vi "SP_REJECTION_Count_DayWise.vi"(8 "error in (no error)":errorcluster) -> (0 "error out":errorcluster)   [LabVIEW 2017]
uses:
  <vilib>/Math Plots/3D Math Plots/3D Pie/3D Pie XCtrl/3D Pie.xctl
  <vilib>/addons/database/Connection.llb/DB Tools Open Connec (Path).vi
  <vilib>/addons/database/Connection.llb/Conn Execute.vi
  <vilib>/addons/database/Recordset.llb/Rec Fetch Recordset Data (R).vi
  <vilib>/addons/database/Recordset.llb/Rec Destroy - Connection.vi
  <vilib>/Math Plots/3D Math Plots/3D Pie/3D Pie Datatype/Public/Plot Helper (Vector).vi
  <vilib>/addons/database/NI_Database_API.lvlib
  <vilib>/Math Plots/3D Math Plots/3D Pie/3D Pie Datatype/3D Pie Datatype.lvclass
panel:
  out "Station list":string[](array[string])
  out "Station size":i32
  in  "Tab Control":enum32{"Data", "Graph"}(tab)
  out "Table":string[][](table)
  out "3D Pie":refnum<class "3D Plot Datatype.lvclass">[](xcontrol)
  in  "To Date":timestamp format="%<%Y-%m-%d>T"
  out "Station Count":i32
  in  "Cancel Button - Archive":bool
  in  "Download 2":bool
  in  "Get Rport 2":bool
  in  "Shift":string(combo)
  in  "Station":string(combo)
  in  "From Date":timestamp format="%<%Y-%m-%d>T"
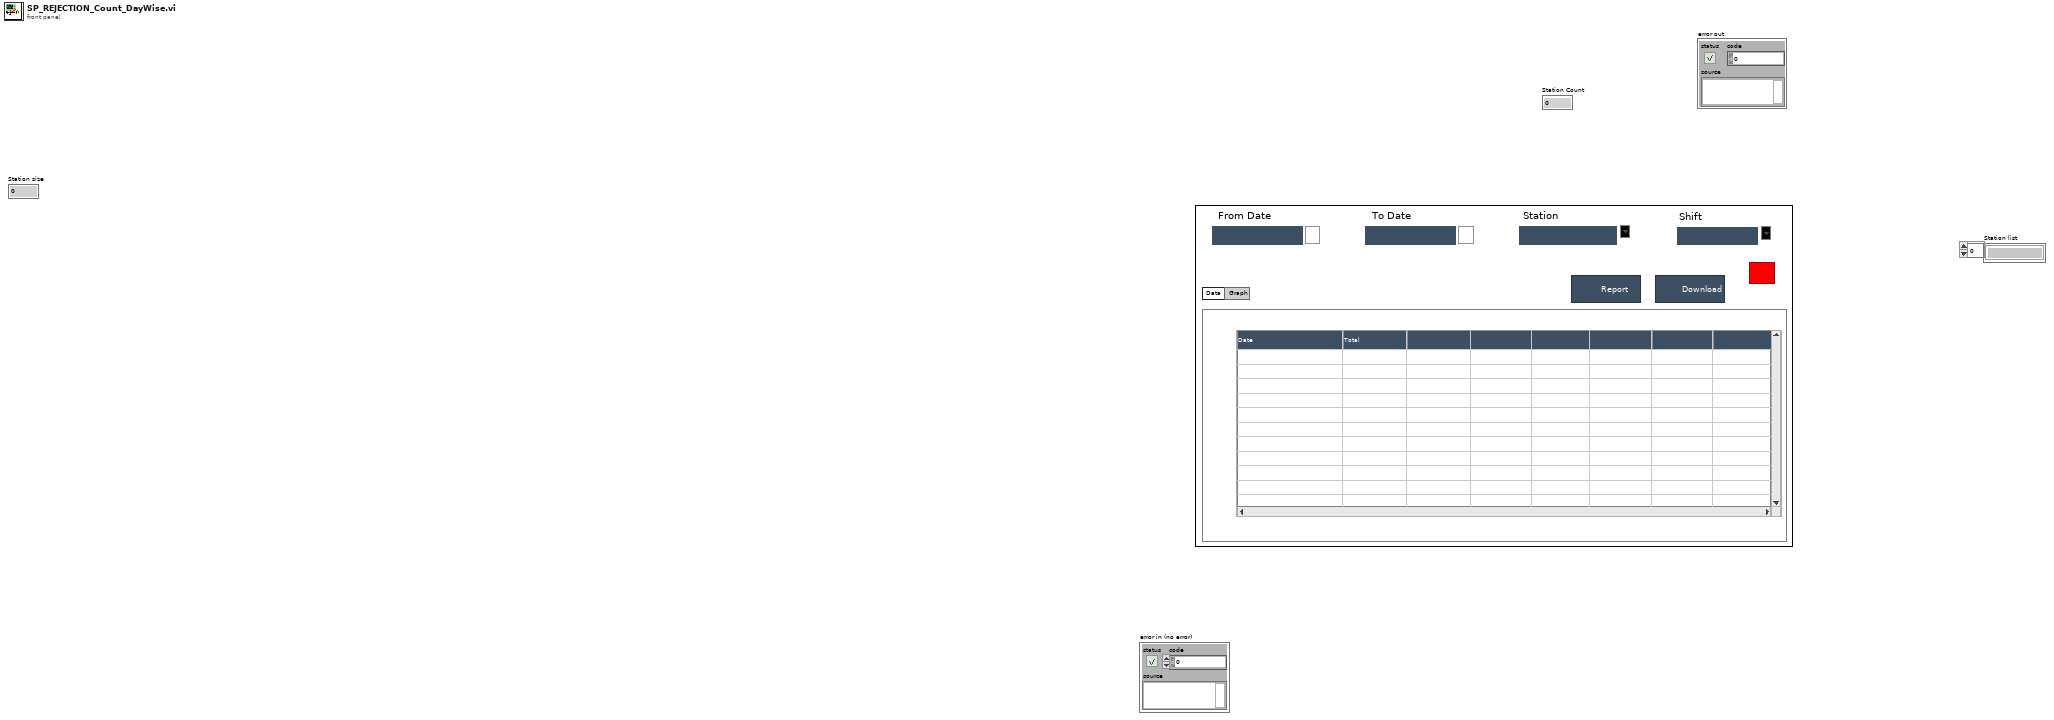
[diagram p1: front panel]
types:
  T1 = typedef "NI_Database_API.lvlib/Conn ObjectReference.ctl" = refnum<k1>
  T2 = typedef "NI_Database_API.lvlib/Rec ObjectReference.ctl" = refnum<k1>
  T3 = enum32{"invalid app kind", "Development System", "Run Time System", "Student Edition", "Embedded LabVIEW", "Evaluation", "Custom"}
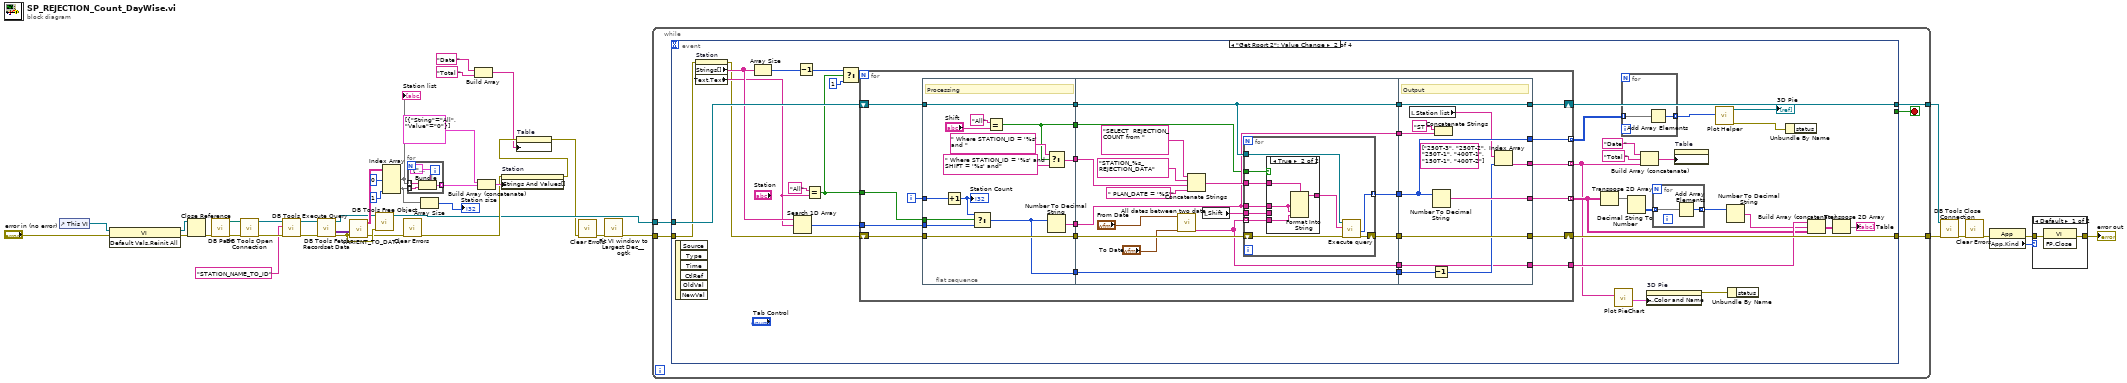
[diagram p0: block diagram]
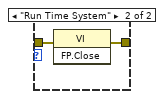
[diagram p2: hidden frame]
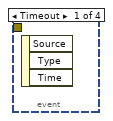
[diagram p3: hidden frame]
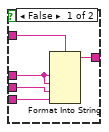
[diagram p4: hidden frame]
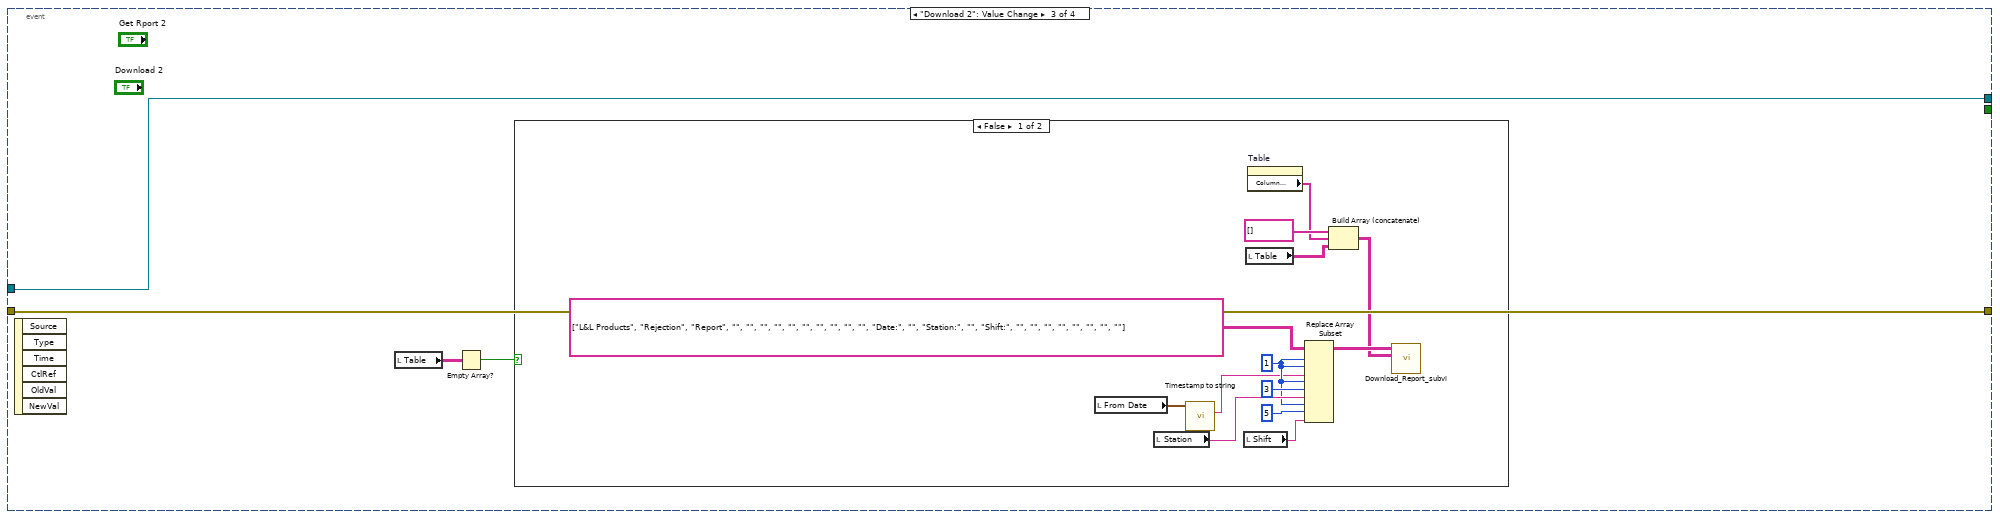
[diagram p5: hidden frame]
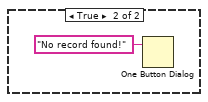
[diagram p6: hidden frame]
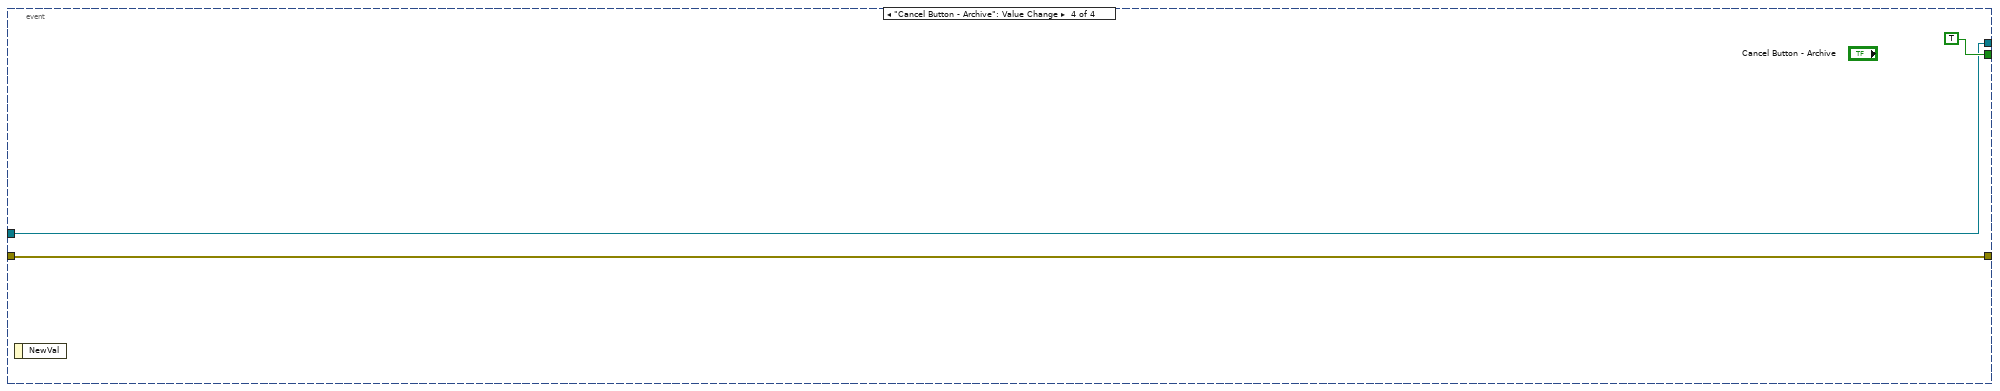
[diagram p7: hidden frame]
diagram:
  n1 = control-ref of="This VI"() -> (w34:refnum<vi>)
  n2 = invoke class="VI" method="Default Vals.Reinit All"(reference=w34, error in="error in (no error)") -> (reference out=w32:refnum<vi>, error out=w33:errorcluster)  [unwired: 1 in, 1 out]
  n3 = Close Reference(reference=w32, error in (no error)=w33) -> (error out=w31:errorcluster)
  n4 = call "DB Path.vi"("error in"=w31) -> ("error out"=w30:errorcluster, "DB Path"=w29:path)  [unwired: 9 in]
  n5 = call-poly <vilib>:"DB Tools Open Connection.vi"("error in (no error)"=w30, "connection information"=w29) -> ("error out"=w18:errorcluster, "connection reference"=w19:T1)  [unwired: 6 in]
  n6 = call-poly <vilib>:"DB Tools Execute Query.vi"("error in (no error)"=w18, "SQL query"="STATION_NAME_TO_ID", "connection reference"=w19) -> ("error out"=w27:errorcluster, "recordset reference"=w28:T2)  [unwired: 5 in]
  n7 = call-poly <vilib>:"DB Tools Fetch Recordset Data.vi"("error in (no error)"=w27, "recordset reference"=w28) -> ("error out"=w22:errorcluster, "recordset data"=w26:variant[][], "recordset reference out"=w20:T2)  [unwired: 3 in]
  n8 = call "VARIENT_TO_DATA.vi"("data"=w26, "error in (no error)"=w22) -> ("Table"=w23:string[][], "error out"=w21:errorcluster)  [unwired: 7 in]
  n9 = call-poly <vilib>:"DB Tools Free Object.vi"("error in (no error)"=w22, "recordset reference"=w20) -> ("connection reference"=w6:T1)  [unwired: 8 in, 1 out]
  n10 = Index Array(array=w23, index (col) #1=0 ("index (row)"), index (col) #2=1 ("index (col)")) -> (element #1=w9:string[], element #2=w12:string[])  [unwired: 2 in]
  "Station list" <- w9
  n11 = call <vilib>:"Clear Errors.vi"("error in (no error)"=w21) -> ("error out"=w14:errorcluster)  [unwired: 5 in, 1 out]
  n12 = for {
    tunnel: w9 -> [w45] mode=indexing
    tunnel: w12 -> [w44] mode=indexing
    tunnel: [w42] -> w13 mode=indexing
    n13 = Bundle(cluster=cluster{"String":string, "Value":string} {"String"="", "Value"=""}, "String"=w45, "Value"=w44) -> (w42:cluster{"String":string, "Value":string})
  }
  n14 = Array Size(array=w12) -> (size(s)=→"Station size":i32)
  n15 = Build Array("Date ", "Total ") -> (w1:string[])
  n16 = Build Array (concatenate)(cluster{"String":string, "Value":string}[] [{"String"="All", "Value"="0"}] ("array"), w13) -> (w16:cluster{"String":string, "Value":string}[])
  n17 = property on="Station" class="CmbBox"(error in=w14, "Strings And Values[]"=w16) -> (error out=w5:errorcluster)  [unwired: 1 in, 1 out]
  n18 = property on="Table" class="Tbl (strict)"(error in=w5, "Column Headers[]"=w1) -> (error out=w4:errorcluster)  [unwired: 1 in, 1 out]
  n19 = call <vilib>:"Clear Errors.vi"("error in (no error)"=w4) -> ("error out"=w10:errorcluster)  [unwired: 5 in, 1 out]
  n20 = call <userlib>:"Fit VI window to Largest Dec__ogtk.vi"("error in (no error)"=w10) -> ("error out"=w7:errorcluster)  [unwired: 5 in, 1 out]
  n21 = while {
    tunnel: w7 -> [w47]
    tunnel: w6 -> [w46]
    tunnel: [w49] -> w37
    tunnel: [w48] -> w36
    stop <- w50 stop-if-true
    n22 = event shown="[1] \"Get Rport 2\": Value Change" {
      selector: _ -> [_ _ _ _]
      dyn-events: _ -> [_ _ _ _]
      timeout: _ -> [_ _ _ _]
      tunnel: w46 -> [_ w82 w173 w189]
      tunnel: [_ _ _ TRUE] -> w50
      tunnel: [_ w80 w172 w188] -> w49
      tunnel: [_ w81 w173 w189] -> w48
      tunnel: w47 -> [_ w52 w172 w188]
      event Timeout {
        n23 = event-data() -> ()  [unwired: 1 in, 3 out]
      }
      event "Get Rport 2": Value Change {
        n24 = event-data() -> ()  [unwired: 1 in, 6 out]
        n25 = property on="Station" class="CmbBox"(error in=w52) -> (error out=w51:errorcluster, "Strings[]"=w61:string[], "Text.Text"=w53:string)  [unwired: 1 in, 1 out]
        n26 = Array Size(array=w61) -> (size(s)=w76:i32)
        n27 = Search 1D Array(1D array=w61, element=w53) -> (index of element=w73:i32)  [unwired: 1 in]
        n28 = Decrement(x=w76) -> (x-1=w75:i32)
        n29 = Equal?(x="All", y=w53) -> (x = y?=w74:bool)
        n30 = Select(t=w75, s=w74, f=1) -> (s? t:f=w78:i32)
        n31 = for {
          N: w78 -> [_]
          shift-right: [w102] -> w81
          shift-left: w82 -> [w109]
          shift-right: [w103] -> w80
          shift-left: w51 -> [w108]
          tunnel: w74 -> [w107]
          tunnel: w73 -> [w106]
          tunnel: [w104] -> w55 mode=indexing
          tunnel: [w94] -> w66 mode=indexing
          tunnel: [w93] -> w69
          tunnel: [w87] -> w57 mode=indexing
          i -> [w105]
          n32 = flat-sequence {
            tunnel: [w120] -> w101
            tunnel: [w121] -> w99
            tunnel: [w123] -> w97
            tunnel: [w122] -> w96
            tunnel: w105 -> [w115]
            tunnel: w106 -> [w116]
            tunnel: w107 -> [w117]
            tunnel: w108 -> [w120]
            tunnel: w109 -> [w121]
            tunnel: [w111] -> w90
            tunnel: [w110] -> w88
            tunnel: w101 -> [w132]
            tunnel: [w131] -> w100
            tunnel: w99 -> [w133]
            tunnel: [w133] -> w98
            tunnel: w97 -> [w137]
            tunnel: w96 -> [w129]
            tunnel: [w130] -> w95
            tunnel: [w129] -> w92
            tunnel: [w128] -> w91
            tunnel: w90 -> [w125]
            tunnel: [w124] -> w89
            tunnel: w88 -> [w124]
            tunnel: [w163] -> w104
            tunnel: w100 -> [w165]
            tunnel: [w165] -> w103
            tunnel: [w169] -> w102
            tunnel: w98 -> [w169]
            tunnel: w95 -> [w161]
            tunnel: [w168] -> w94
            tunnel: [w160] -> w93
            tunnel: w92 -> [w167]
            tunnel: w91 -> [w160]
            tunnel: w89 -> [w164]
            tunnel: [w161] -> w87
            frame #0 {
              # "Processing"
              n33 = Increment(x=w115) -> (x+1=w114:i32)
              "Station Count" <- w114
              n34 = Select(t=w114, s=w117, f=w116) -> (s? t:f=w110:i32)
              n35 = Equal?(x="All", y="Shift") -> (x = y?=w111:bool)
              n36 = Select(t=" Where STATION_ID = '%s' and " ("format string"), s=w111, f=" Where STATION_ID = '%s' and SHIFT = '%s' and" ("format string")) -> (s? t:f=w123:string)
              n37 = Number To Decimal String(number=w110) -> (decimal integer string=w122:string)  [unwired: 1 in]
            }
            frame #1 {
              n38 = call "All dates between two date.vi"("To Date"="To Date", "From Date"="From Date") -> ("All Days (String)"=w128:string[])  [unwired: 8 in, 1 out]
              n39 = Concatenate Strings("SELECT  REJECTION_COUNT from " ("format string"), "STATION_%s_REJECTION_DATA", w137, " PLAN_DATE = '%S'" ("string")) -> (w135:string)
              n40 = local read "Shift"() -> (w134:string)
              n41 = for {
                tunnel: w125 -> [w149]
                tunnel: w135 -> [w148]
                tunnel: w129 -> [w147]
                tunnel: w134 -> [w146]
                tunnel: w128 -> [w145] mode=indexing
                tunnel: w133 -> [w143]
                shift-right: [w141] -> w131
                shift-left: w132 -> [w142]
                tunnel: [w140] -> w130 mode=indexing
                n42 = case shown="True" w149 {
                  tunnel: w148 -> [w154 w158]
                  tunnel: w147 -> [w153 w157]
                  tunnel: w146 -> [w152 _]
                  tunnel: w145 -> [w151 w156]
                  tunnel: [w150 w155] -> w144
                  frame False {
                    n43 = Format Into String(format string=w154, w153, w153, w152, w151) -> (resulting string=w150:string)  [unwired: 2 in, 1 out]
                  }
                  frame True {
                    n44 = Format Into String(format string=w158, w157, w157, w156) -> (resulting string=w155:string)  [unwired: 2 in, 1 out]
                  }
                }
                n45 = call "Execute query.vi"("error in (no error)"=w142, "String"=w144, "connection reference"=w143) -> ("error out"=w141:errorcluster, "Production Count"=w140:i32)  [unwired: 3 in, 4 out]
              }
            }
            frame #2 {
              (unwired) string[] ["250T-3", "250T-2", "250T-1", "400T-1", "150T-1", "400T-2"]
              # "Output"
              n46 = local read "Station list"() -> (w159:string[])
              n47 = Decrement(x=w164) -> (x-1=w162:i32)
              n48 = Number To Decimal String(number=w161) -> (decimal integer string=w168:string[])  [unwired: 1 in]
              n49 = Concatenate Strings("ST " ("string"), w167) -> ()  [unwired: 1 out]
              n50 = Index Array(array=w159, index=w162) -> (element=w163:string)
            }
          }
        }
        n51 = Transpose 2D Array(2D array=w66) -> (transposed array=w65:string[][])
        n52 = call "Plot PieChart.vi"("Label"=w55) -> ("Labelling"=w56:cluster{dbl, "String":string}[])  [unwired: 10 in]
        n53 = for {
          tunnel: w57 -> [w84] mode=indexing
          tunnel: [w83] -> w58 mode=indexing
          n54 = Add Array Elements(numeric array=w84) -> (sum=w83:i32)
        }
        n55 = Decimal String To Number(string=w65) -> (number=w64:i32[][])  [unwired: 2 in, 1 out]
        n56 = Build Array (concatenate)("Date ", "Total ", w55) -> (w72:string[])
        n57 = property on="3D Pie" class="3D Pie (strict)"("Plot Specific:Color and Name"=w56) -> (error out=w54:errorcluster)  [unwired: 2 in, 1 out]
        n58 = for {
          tunnel: w64 -> [w86] mode=indexing
          tunnel: [w85] -> w63 mode=indexing
          n59 = Add Array Elements(numeric array=w86) -> (sum=w85:i32)
        }
        n60 = property on="Table" class="Tbl (strict)"("Column Headers[]"=w72) -> ()  [unwired: 2 in, 2 out]
        n61 = call-poly <vilib>:"Plot Helper.vi"("x vector"=w58) -> ("error out"=w59:errorcluster, "3D Plot lvclass Array out"=→"3D Pie":refnum<class "3D Plot Datatype.lvclass">[])  [unwired: 2 in, 7 out]
        n62 = Number To Decimal String(number=w63) -> (decimal integer string=w62:string[])  [unwired: 1 in]
        n63 = Unbundle By Name(w54) -> ()  [unwired: 1 out]
        n64 = Unbundle By Name(w59) -> ()  [unwired: 1 out]
        n65 = Build Array (concatenate)(w69, w62, w66) -> (w71:string[][])
        n66 = Transpose 2D Array(2D array=w71) -> (transposed array=→"Table":string[][])
      }
      event "Download 2": Value Change {
        n67 = event-data() -> ()  [unwired: 1 in, 6 out]
        n68 = local read "Table"() -> (w171:string[][])
        n69 = Empty Array?(array=w171) -> (empty?=w170:bool)
        n70 = case shown="False" w170 {
          frame False {
            w182 = 1 ("index (row)")
            n71 = local read "From Date"() -> (w179:timestamp)
            n72 = local read "Station"() -> (w183:string)
            n73 = call "Timestamp to string.vi"("time stamp"=w179) -> ("Date"=w178:string)  [unwired: 8 in, 2 out]
            n74 = local read "Shift"() -> (w180:string)
            n75 = local read "Table"() -> (w177:string[][])
            n76 = property on="Table" class="Tbl (strict)"() -> ("Column Headers[]"=w174:string[])  [unwired: 2 in, 2 out]
            n77 = Replace Array Subset(array=string[][] [["L&L Products", "Rejection", "Report", "", "", "", "", "", "", "", "", "", ""], ["Date:", "", "Station:", "", "Shift:", "", "", "", "", "", "", "", ""]] ("Column Header Strings[]"), new element #1=w178, index (row) #1=w182, index (col) #1=w182, new element #2=w183, index (row) #2=w182, index (col) #2=3 ("disabled index (col)"), new element #3=w180, index (row) #3=w182, index (col) #3=5 ("disabled index (col)")) -> (w185:string[][])
            n78 = Build Array (concatenate)(string[] [] ("element"), w174, w177) -> (w176:string[][])
            n79 = call "Download_Report_subvi.vi"("Value"=w176, "Column Header Strings[]"=w185) -> ()  [unwired: 9 in, 1 out]
          }
          frame True {
            n80 = One Button Dialog(message="No record found!") -> ()  [unwired: 1 in, 1 out]
          }
        }
      }
      event "Cancel Button - Archive": Value Change {
        n81 = event-data() -> ()  [unwired: 1 in, 1 out]
      }
    }
  }
  n82 = call <vilib>:"DB Tools Close Connection.vi"("error in (no error)"=w37, "connection reference"=w36) -> ("error out"=w39:errorcluster)  [unwired: 5 in]
  n83 = call <vilib>:"Clear Errors.vi"("error in (no error)"=w39) -> ("error out"=w38:errorcluster)  [unwired: 5 in, 1 out]
  n84 = property class="App"(error in=w38) -> (error out=w40:errorcluster, "App.Kind"=w41:T3)  [unwired: 1 in, 1 out]
  n85 = case shown="Default" w41 {
    tunnel: w40 -> [w192 w194]
    tunnel: [w191 w193] -> w35
    frame Default {
      n86 = invoke class="VI" method="FP.Close"(error in=w192) -> (error out=w191:errorcluster)  [unwired: 2 in, 2 out]
    }
    frame "Run Time System" {
      n87 = invoke class="VI" method="FP.Close"(error in=w194) -> (error out=w193:errorcluster)  [unwired: 2 in, 2 out]
    }
  }
  "error out" <- w35
